vi "LoadLogMessageViewer.vi"(7 "Messages viewer":refnum<vi>, 8 "error In":errorcluster, 11 "MessageArray":T1[](array[typedef])) -> (0 "error out":errorcluster)   [LabVIEW 2011]
uses:
  030 - EVENTS/03 - ToMessageHandlerProcess/ToMessageHandlerEvent.ctl
  030 - EVENTS/03 - ToMessageHandlerProcess/enumMessageCriticity.ctl
  <vilib>/Utility/miscctls.llb/LVRowAndColumnTypeDef.ctl
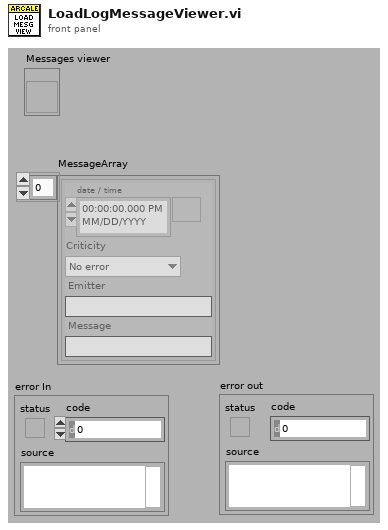
[diagram p1: front panel]
types:
  T1 = typedef "ToMessageHandlerEvent.ctl" = cluster{"date / time":timestamp, "Criticity":T2, "Emitter":string, "Message":string}
  T2 = typedef "enumMessageCriticity.ctl" = enum16{"No error", "Info", "Warning", "Error", "Fatal error"}
  T3 = typedef "LVRowAndColumnTypeDef.ctl" = cluster{"Row":i32, "Column":i32}
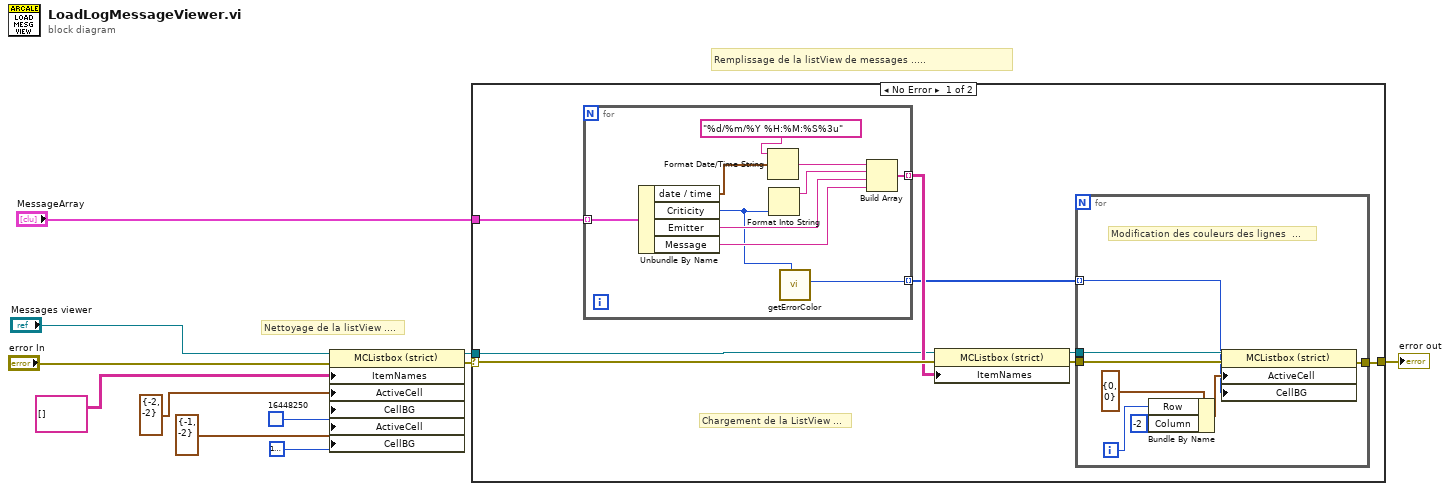
[diagram p0: block diagram]
diagram:
  # "Nettoyage de la listView ...."
  # "Remplissage de la listView de messages ....."
  n1 = property class="MCListbox (strict)"(reference="Messages viewer", error in="error In", "ItemNames"=string[][] [] ("Item Names"), "ActiveCell"=T3 {"Row"=-2, "Column"=-2} ("Active Cell:Active Cell"), "CellBG"=u32 16448250, "ActiveCell"=T3 {"Row"=-1, "Column"=-2} ("Active Cell:Active Cell"), "CellBG"=u32 16777238) -> (reference out=w9:refnum<vi>, error out=w2:errorcluster)
  n2 = case shown="No Error" w2 {
    selector: w2 -> [w19 w38]
    tunnel: [w13 w38] -> w11
    tunnel: w9 -> [w17 _]
    tunnel: "MessageArray" -> [w12 _]
    frame No Error {
      # "Chargement de la ListView ..."
      n3 = for {
        tunnel: w12 -> [w37] mode=indexing
        tunnel: [w30] -> w18 mode=indexing
        tunnel: [w28] -> w14 mode=indexing
        n4 = Unbundle By Name(w37) -> ("date / time"=w36:timestamp, "Criticity"=w29:T2, "Emitter"=w32:string, "Message"=w31:string)
        n5 = Format Date/Time String(time format string (%c)="%d/%m/%Y %H:%M:%S%3u", seconds (now)=w36) -> (date/time string=w34:string)  [unwired: 1 in]
        n6 = Format Into String(w29) -> (resulting string=w33:string)  [unwired: 3 in, 1 out]
        n7 = call "getErrorColor.vi"("Criticity"=w29) -> ("errorColor"=w28:u32)  [unwired: 9 in, 1 out]
        n8 = Build Array(w34, w33, w32, w31) -> (w30:string[])
      }
      n9 = property class="MCListbox (strict)"(reference=w17, error in=w19, "ItemNames"=w18) -> (reference out=w15:refnum<vi>, error out=w16:errorcluster)
      n10 = for {
        tunnel: w16 -> [w27]
        tunnel: w15 -> [w26]
        tunnel: w14 -> [w20] mode=indexing
        tunnel: [w21] -> w13
        i -> [w22]
        # "Modification des couleurs des lignes  ..."
        n11 = Bundle By Name(cluster=T3 {"Row"=0, "Column"=0} ("Active Cell:Active Cell"), "Row"=w22, "Column"=-2) -> (w24:T3)
        n12 = property class="MCListbox (strict)"(reference=w26, error in=w27, "ActiveCell"=w24, "CellBG"=w20) -> (error out=w21:errorcluster)  [unwired: 1 out]
      }
    }
    frame Error {
    }
  }
  "error out" <- w11
